vi "DAQ - SubVI.vi"(11 "array":dbl[](array[numeric])) -> (3 "output array":dbl[](array[numeric]))   [LabVIEW 2013]
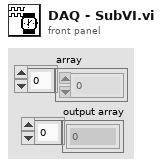
[diagram p1: front panel]
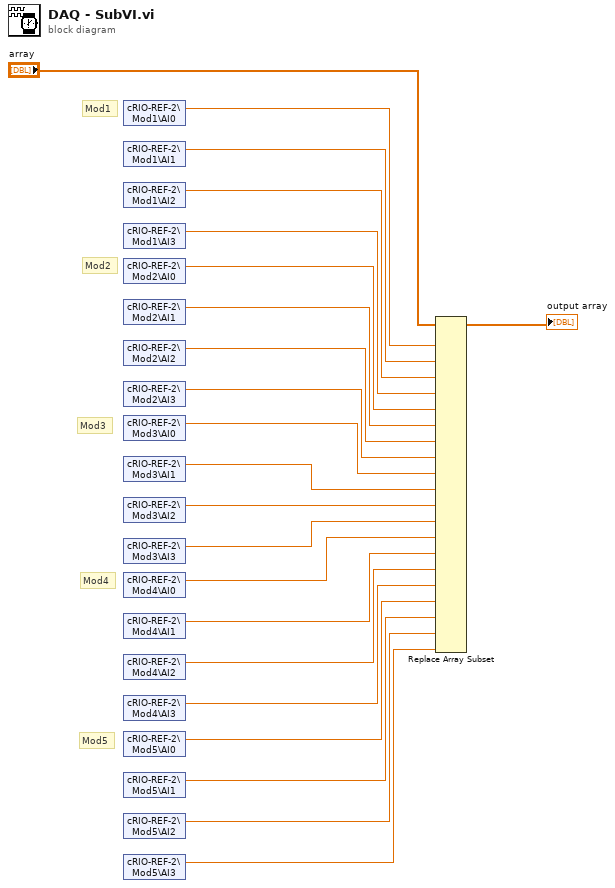
[diagram p0: block diagram]
diagram:
  # "Mod5"
  # "Mod4"
  # "Mod3"
  # "Mod2"
  # "Mod1"
  n1 = shared-variable "cRIO-REF-2\\Mod1\\AI0"() -> (w22:dbl)  [unwired: 1 in, 1 out]
  n2 = shared-variable "cRIO-REF-2\\Mod1\\AI1"() -> (w21:dbl)  [unwired: 1 in, 1 out]
  n3 = shared-variable "cRIO-REF-2\\Mod1\\AI2"() -> (w20:dbl)  [unwired: 1 in, 1 out]
  n4 = shared-variable "cRIO-REF-2\\Mod1\\AI3"() -> (w19:dbl)  [unwired: 1 in, 1 out]
  n5 = shared-variable "cRIO-REF-2\\Mod2\\AI0"() -> (w18:dbl)  [unwired: 1 in, 1 out]
  n6 = shared-variable "cRIO-REF-2\\Mod2\\AI1"() -> (w17:dbl)  [unwired: 1 in, 1 out]
  n7 = shared-variable "cRIO-REF-2\\Mod2\\AI2"() -> (w16:dbl)  [unwired: 1 in, 1 out]
  n8 = shared-variable "cRIO-REF-2\\Mod2\\AI3"() -> (w15:dbl)  [unwired: 1 in, 1 out]
  n9 = shared-variable "cRIO-REF-2\\Mod3\\AI0"() -> (w14:dbl)  [unwired: 1 in, 1 out]
  n10 = shared-variable "cRIO-REF-2\\Mod3\\AI1"() -> (w13:dbl)  [unwired: 1 in, 1 out]
  n11 = shared-variable "cRIO-REF-2\\Mod3\\AI2"() -> (w12:dbl)  [unwired: 1 in, 1 out]
  n12 = shared-variable "cRIO-REF-2\\Mod3\\AI3"() -> (w11:dbl)  [unwired: 1 in, 1 out]
  n13 = shared-variable "cRIO-REF-2\\Mod4\\AI0"() -> (w10:dbl)  [unwired: 1 in, 1 out]
  n14 = shared-variable "cRIO-REF-2\\Mod4\\AI1"() -> (w9:dbl)  [unwired: 1 in, 1 out]
  n15 = shared-variable "cRIO-REF-2\\Mod4\\AI2"() -> (w8:dbl)  [unwired: 1 in, 1 out]
  n16 = shared-variable "cRIO-REF-2\\Mod4\\AI3"() -> (w7:dbl)  [unwired: 1 in, 1 out]
  n17 = shared-variable "cRIO-REF-2\\Mod5\\AI0"() -> (w6:dbl)  [unwired: 1 in, 1 out]
  n18 = shared-variable "cRIO-REF-2\\Mod5\\AI1"() -> (w5:dbl)  [unwired: 1 in, 1 out]
  n19 = shared-variable "cRIO-REF-2\\Mod5\\AI2"() -> (w4:dbl)  [unwired: 1 in, 1 out]
  n20 = shared-variable "cRIO-REF-2\\Mod5\\AI3"() -> (w3:dbl)  [unwired: 1 in, 1 out]
  n21 = Replace Array Subset(array="array", new element #1=w22, new element #2=w21, new element #3=w20, new element #4=w19, new element #5=w18, new element #6=w17, new element #7=w16, new element #8=w15, new element #9=w14, new element #10=w13, new element #11=w12, new element #12=w11, new element #13=w10, new element #14=w9, new element #15=w8, new element #16=w7, new element #17=w6, new element #18=w5, new element #19=w4, new element #20=w3) -> (→"output array":dbl[])  [unwired: 20 in]
